vi "Create Nominal Ingestion Config Response.vi"() -> (2 "output cluster":T1)   [LabVIEW 2024]
uses:
  Private/Typedefs/Messages/JSON Response.ctl
  Private/Typedefs/Messages/Create Ingestion Config Response.ctl
  Sift Client.lvlib
panel:
  in  "Create Ingestion Config Reponse":T2
  in  "JSON Response":T1
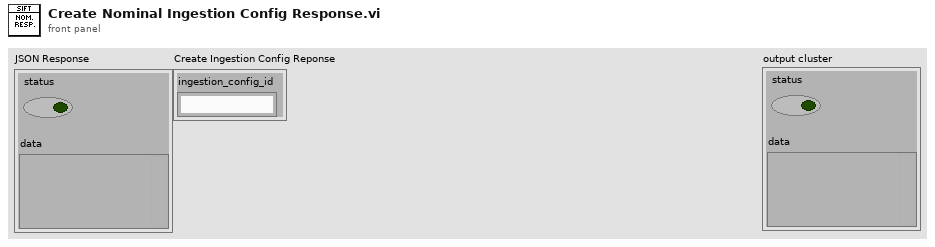
[diagram p1: front panel]
types:
  T1 = typedef "Sift Client.lvlib/JSON Response.ctl" = cluster{"status":bool, "data":variant}
  T2 = typedef "Sift Client.lvlib/Create Ingestion Config Response.ctl" = cluster{"ingestion_config_id":string}
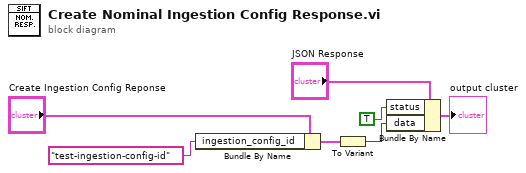
[diagram p0: block diagram]
diagram:
  n1 = Bundle By Name(cluster="Create Ingestion Config Reponse", "ingestion_config_id"="test-ingestion-config-id") -> (w3:T2)
  n2 = To Variant(anything=w3) -> (Variant=w2:variant)
  n3 = Bundle By Name(cluster="JSON Response", "status"=TRUE, "data"=w2) -> (→"output cluster":T1)
